vi "Gear Delivery Logging.vi"   [LabVIEW 2016]
uses:
  Robot Global Data.vi
  Gear Delivery Logging Values.vi
types:
  T1 = typedef "WPI_DriverStationRobotMode2.ctl" = enum16{"Autonomous Disabled", "Autonomous Enabled", "Teleop Disabled", "Teleop Enabled", "Disconnected", "Finish", "Test Disabled", "Test Enabled", "Emergency Stopped"}
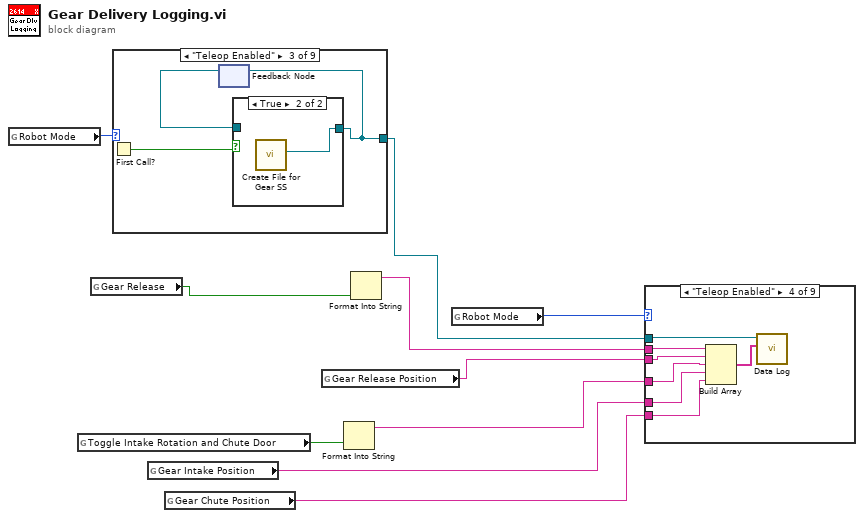
[diagram p0: block diagram]
diagram:
  n1 = global read "Robot Global Data.vi" "Robot Mode"() -> (w8:T1)
  n2 = global read "Gear Delivery Logging Values.vi" "Toggle Intake Rotation and Chute Door"() -> (w3:bool)
  n3 = global read "Gear Delivery Logging Values.vi" "Gear Release"() -> (w4:bool)
  n4 = case shown="\"Teleop Enabled\"" w8 {
    tunnel: [_ _ w11 _ _ _ _ _ _] -> w7
    frame "Autonomous Enabled" {
    }
    frame "Teleop Disabled", Default {
    }
    frame "Teleop Enabled" {
      n5 = First Call?() -> (First Call?: T/F=w13:bool)
      n6 = feedback #1() -> (w12:refnum<file>)  [unwired: 1 in]
      n7 = case shown="True" w13 {
        tunnel: [w14 w15] -> w11
        tunnel: w12 -> [w14 _]
        frame False {
        }
        frame True {
          n8 = call "Create File for Gear SS.vi"() -> ("File Reference Out"=w15:refnum<file>)  [unwired: 11 in]
        }
      }
      n9 = feedback-in #1(w11) -> ()
    }
    frame "Disconnected" {
    }
    frame "Finish" {
    }
    frame "Test Disabled" {
    }
    frame "Test Enabled" {
    }
    frame "Emergency Stopped" {
    }
    frame "Autonomous Disabled" {
    }
  }
  n10 = global read "Gear Delivery Logging Values.vi" "Gear Intake Position"() -> (w2:string)
  n11 = global read "Gear Delivery Logging Values.vi" "Gear Chute Position"() -> (w1:string)
  n12 = global read "Gear Delivery Logging Values.vi" "Gear Release Position"() -> (w5:string)
  n13 = Format Into String(w3) -> (resulting string=w9:string)  [unwired: 3 in, 1 out]
  n14 = Format Into String(w4) -> (resulting string=w10:string)  [unwired: 3 in, 1 out]
  n15 = global read "Robot Global Data.vi" "Robot Mode"() -> (w6:T1)
  n16 = case shown="\"Teleop Enabled\"" w6 {
    tunnel: w10 -> [_ _ _ w20 _ _ _ _ _]
    tunnel: w9 -> [_ _ _ w19 _ _ _ _ _]
    tunnel: w7 -> [_ _ _ w21 _ _ _ _ _]
    tunnel: w5 -> [_ _ _ w18 _ _ _ _ _]
    tunnel: w2 -> [_ _ _ w17 _ _ _ _ _]
    tunnel: w1 -> [_ _ _ w16 _ _ _ _ _]
    frame "Autonomous Disabled", Default {
    }
    frame "Autonomous Enabled" {
    }
    frame "Teleop Disabled" {
    }
    frame "Teleop Enabled" {
      n17 = Build Array(w20, w18, w19, w17, w16) -> (w22:string[])
      n18 = call "Data Log.vi"("Data In"=w22, "File Reference In"=w21) -> ()  [unwired: 9 in, 1 out]
    }
    frame "Disconnected" {
    }
    frame "Finish" {
    }
    frame "Test Disabled" {
    }
    frame "Test Enabled" {
    }
    frame "Emergency Stopped" {
    }
  }
